vi "How to use in host.vi"(9 "element":string) -> (1 "2D Picture":picture, 11 "Select Part":u16(ring) items=["P1.JPG", "P10.JPG", "P11.JPG", "P12.JPG", "P13.JPG", "P14.JPG", "P15.JPG", "P2.JPG", "P3.JPG", "P4.JPG", "P5.JPG", "P6.JPG", "P8.JPG", "P9.JPG"])   [LabVIEW 2015]
uses:
  Galobal variable_TI.vi
panel:
  out "error out":errorcluster
  out "empty?":bool
  in  "stop":bool
  out "filenames":string[](array[string])
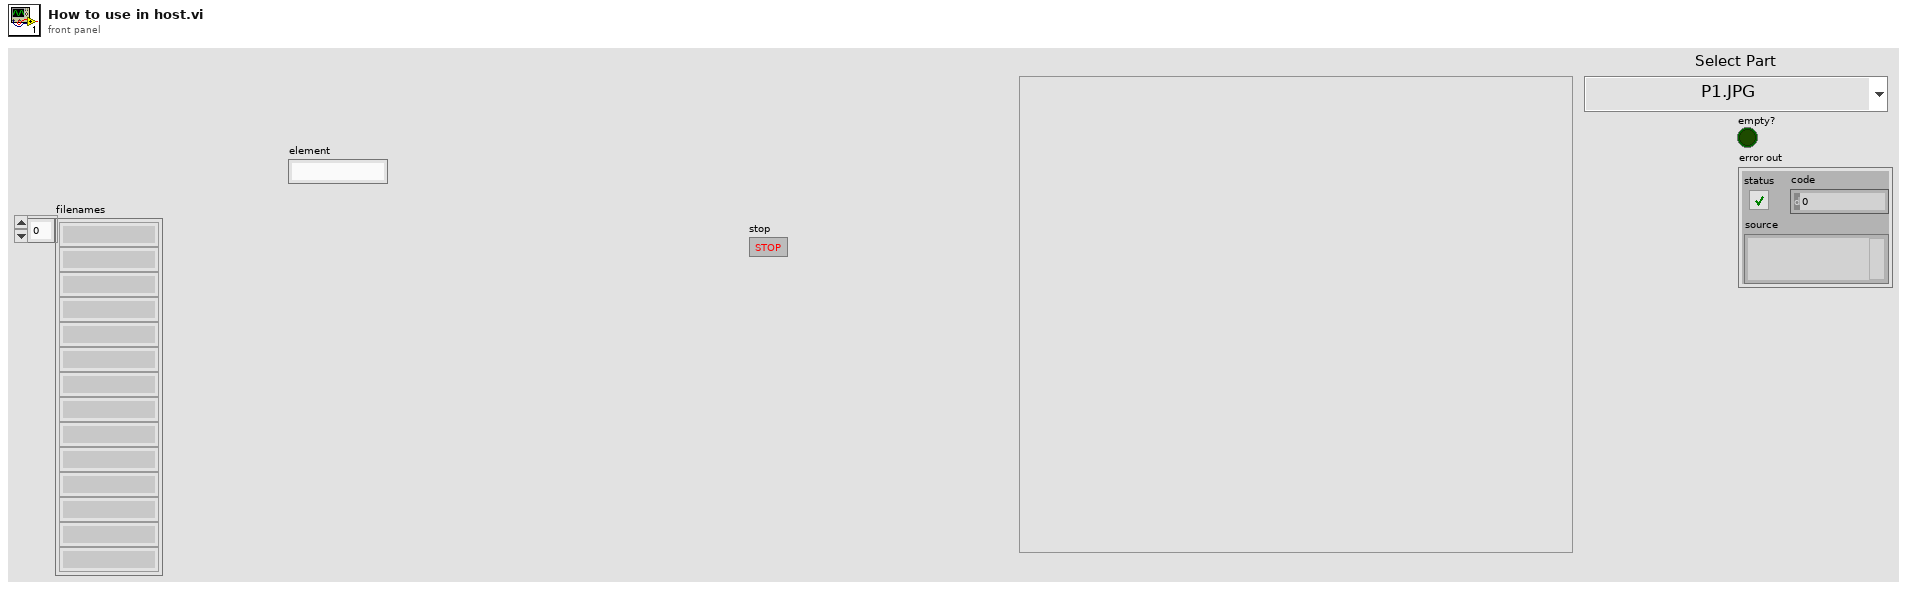
[diagram p1: front panel]
types:
  T1 = typedef "imagedata.ctl" = cluster{"image type":i32, "image depth":i32, "image":u8[], "mask":u8[], "colors":u32[], "Rectangle":cluster{"left":i16, "top":i16, "right":i16, "bottom":i16}}
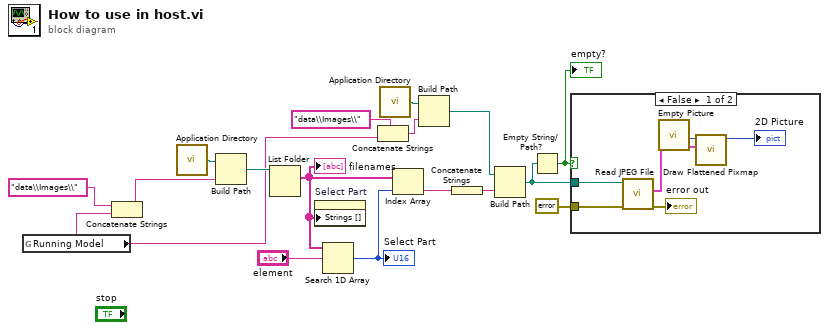
[diagram p0: block diagram]
diagram:
  n1 = global read "Galobal variable_TI.vi" "Running Model"() -> (w2:string)
  n2 = Concatenate Strings("data\\Images\\" ("name or relative path"), w2) -> (w5:string)
  n3 = call <vilib>:"Application Directory.vi"() -> ("Application Directory"=w17:path)
  n4 = Build Path(base path=w17, name or relative path=w5) -> (appended path=w16:path)
  n5 = List Folder(path=w16) -> (filenames=w15:string[])  [unwired: 3 in, 3 out]
  "filenames" <- w15
  n6 = property on="Select Part" class="Ring (strict)"("Strings []"=w15) -> ()  [unwired: 2 in, 2 out]
  n7 = Search 1D Array(1D array=w15, element="element") -> (index of element=w14:i32)  [unwired: 1 in]
  "Select Part" <- w14
  n8 = Concatenate Strings("data\\Images\\" ("name or relative path"), w2) -> (w1:string)
  n9 = call <vilib>:"Application Directory.vi"() -> ("Application Directory"=w11:path)
  n10 = Index Array(array=w15, index=w14) -> (element=w4:string)
  n11 = Build Path(base path=w11, name or relative path=w1) -> (appended path=w10:path)
  n12 = Concatenate Strings(w4) -> (w12:string)
  n13 = Build Path(base path=w10, name or relative path=w12) -> (appended path=w9:path)
  n14 = Empty String/Path?(string/path=w9) -> (empty?=w8:bool)
  "empty?" <- w8
  n15 = case shown="False" w8 {
    tunnel: w9 -> [w20 _]
    tunnel: errorcluster {"status"=FALSE, "code"=0, "source"=""} ("error in (no error)") -> [w19 _]
    frame False {
      n16 = call <vilib>:"Read JPEG File.vi"("error in (no error)"=w19, "path to JPEG file"=w20) -> ("error out"=→"error out":errorcluster, "image data"=w22:T1)  [unwired: 7 in, 1 out]
      n17 = call "Empty Picture"() -> ("empty picture"=w23:picture)
      n18 = call <vilib>:"Draw Flattened Pixmap.vi"("image data"=w22, "picture"=w23) -> ("new picture"=→"2D Picture":picture)  [unwired: 7 in]
    }
    frame True {
    }
  }
